vi "Estimate_State-Space_Model_from_FRFs_Parameter_Adjustment_v3.vi"() -> ()   [LabVIEW 2022 SP3]
doc: "This example demonstrates how to use frequency-domain data to estimate a state-space model. \n\n<B>Instructions:</B>\n1) Run this VI.\n2) Observe how the simulated frequency response matches the measured frequency response.\n3) Change the orders of the models, and observe how these changes affect the estimation error."
uses:
  WhiteNoise.ctl
  <vilib>/addons/System Identification/Model Typedefs.llb/SI Pole-Zero Plot.ctl
  <vilib>/addons/System Identification/Frequency Domain Estimation.llb/SI Estimate Discrete State-Space Model from FRF (SISO Arbitrary).vi
  <vilib>/addons/System Identification/Model Analysis.llb/SI Model Simulation (SISO Waveform).vi
  <vilib>/measure/maspectr.llb/FFT Spectrum (Mag-Phase) for 1 Chan.vi
  <vilib>/addons/System Identification/NI_SysID.lvlib
  <vilib>/addons/System Identification/Model Management Subs.llb/SI Get Order of SS Model (SISO).vi
  <vilib>/measure/NI_MABase.lvlib
  <vilib>/measure/NI_MAPro.lvlib
panel:
  out "Phase 2":cluster{"f0":dbl, "df":dbl, "phase":dbl[]}(graph)
  out "Mag 2":cluster{"f0":dbl, "df":dbl, "magnitude":dbl[]}(graph)
  out "Waveform Graph 2":waveform(dbl)(graph)
  out "Waveform Graph":waveform(dbl)(graph)
  in  "?":enum32{"White Noise", "Harmonic"}(tab)
  in  "Cluster":T2={"Seed"=0.0, "Standard Deviation"=0.2, "Reset"=FALSE, "Iterator"=1.0} {"Standard Deviation" format="%0.2p"}
  in  "Cluster 2":T3={"Iterator"=1.0, "Waveform Type"=0, "Frequency"=10.0, "Amplitude"=0.5} {"Frequency" format="%0.2p"; "Waveform Type" items=["Sine Wave", "Triangle Wave", "Square Wave", "Sawtooth Wave"]; "Amplitude" format="%0.2p"}
  out "sampling rate (Hz)":dbl
  out "model":picture
  out "number of states":i32
  out "Phase Error":cluster{dbl[], dbl[]}(graph)
  in  "confidence level (%)":dbl=99.0 format="%_2f"
  out "pole-zero plot":T4
  in  "name or relative path":path=path "C:/Users/LAV-UFSC/OneDrive - UFSC/Documents/LAV - TCC/Dados-Experimentos/25-04/frf_2.txt"
  in  "noise subspace (%)":dbl=78.0
  in  "FRF format":T5={"dB on? (F)"=FALSE, "unwrap phase? (F)"=FALSE, "convert to degree? (F)"=TRUE}
  out "Phase Response":cluster{"frequency":dbl[], "amplitude":dbl[]}[](graph)
  out "Magnitude Response":cluster{"frequency":dbl[], "amplitude":dbl[]}[](graph)
  in  "Order":i32=9
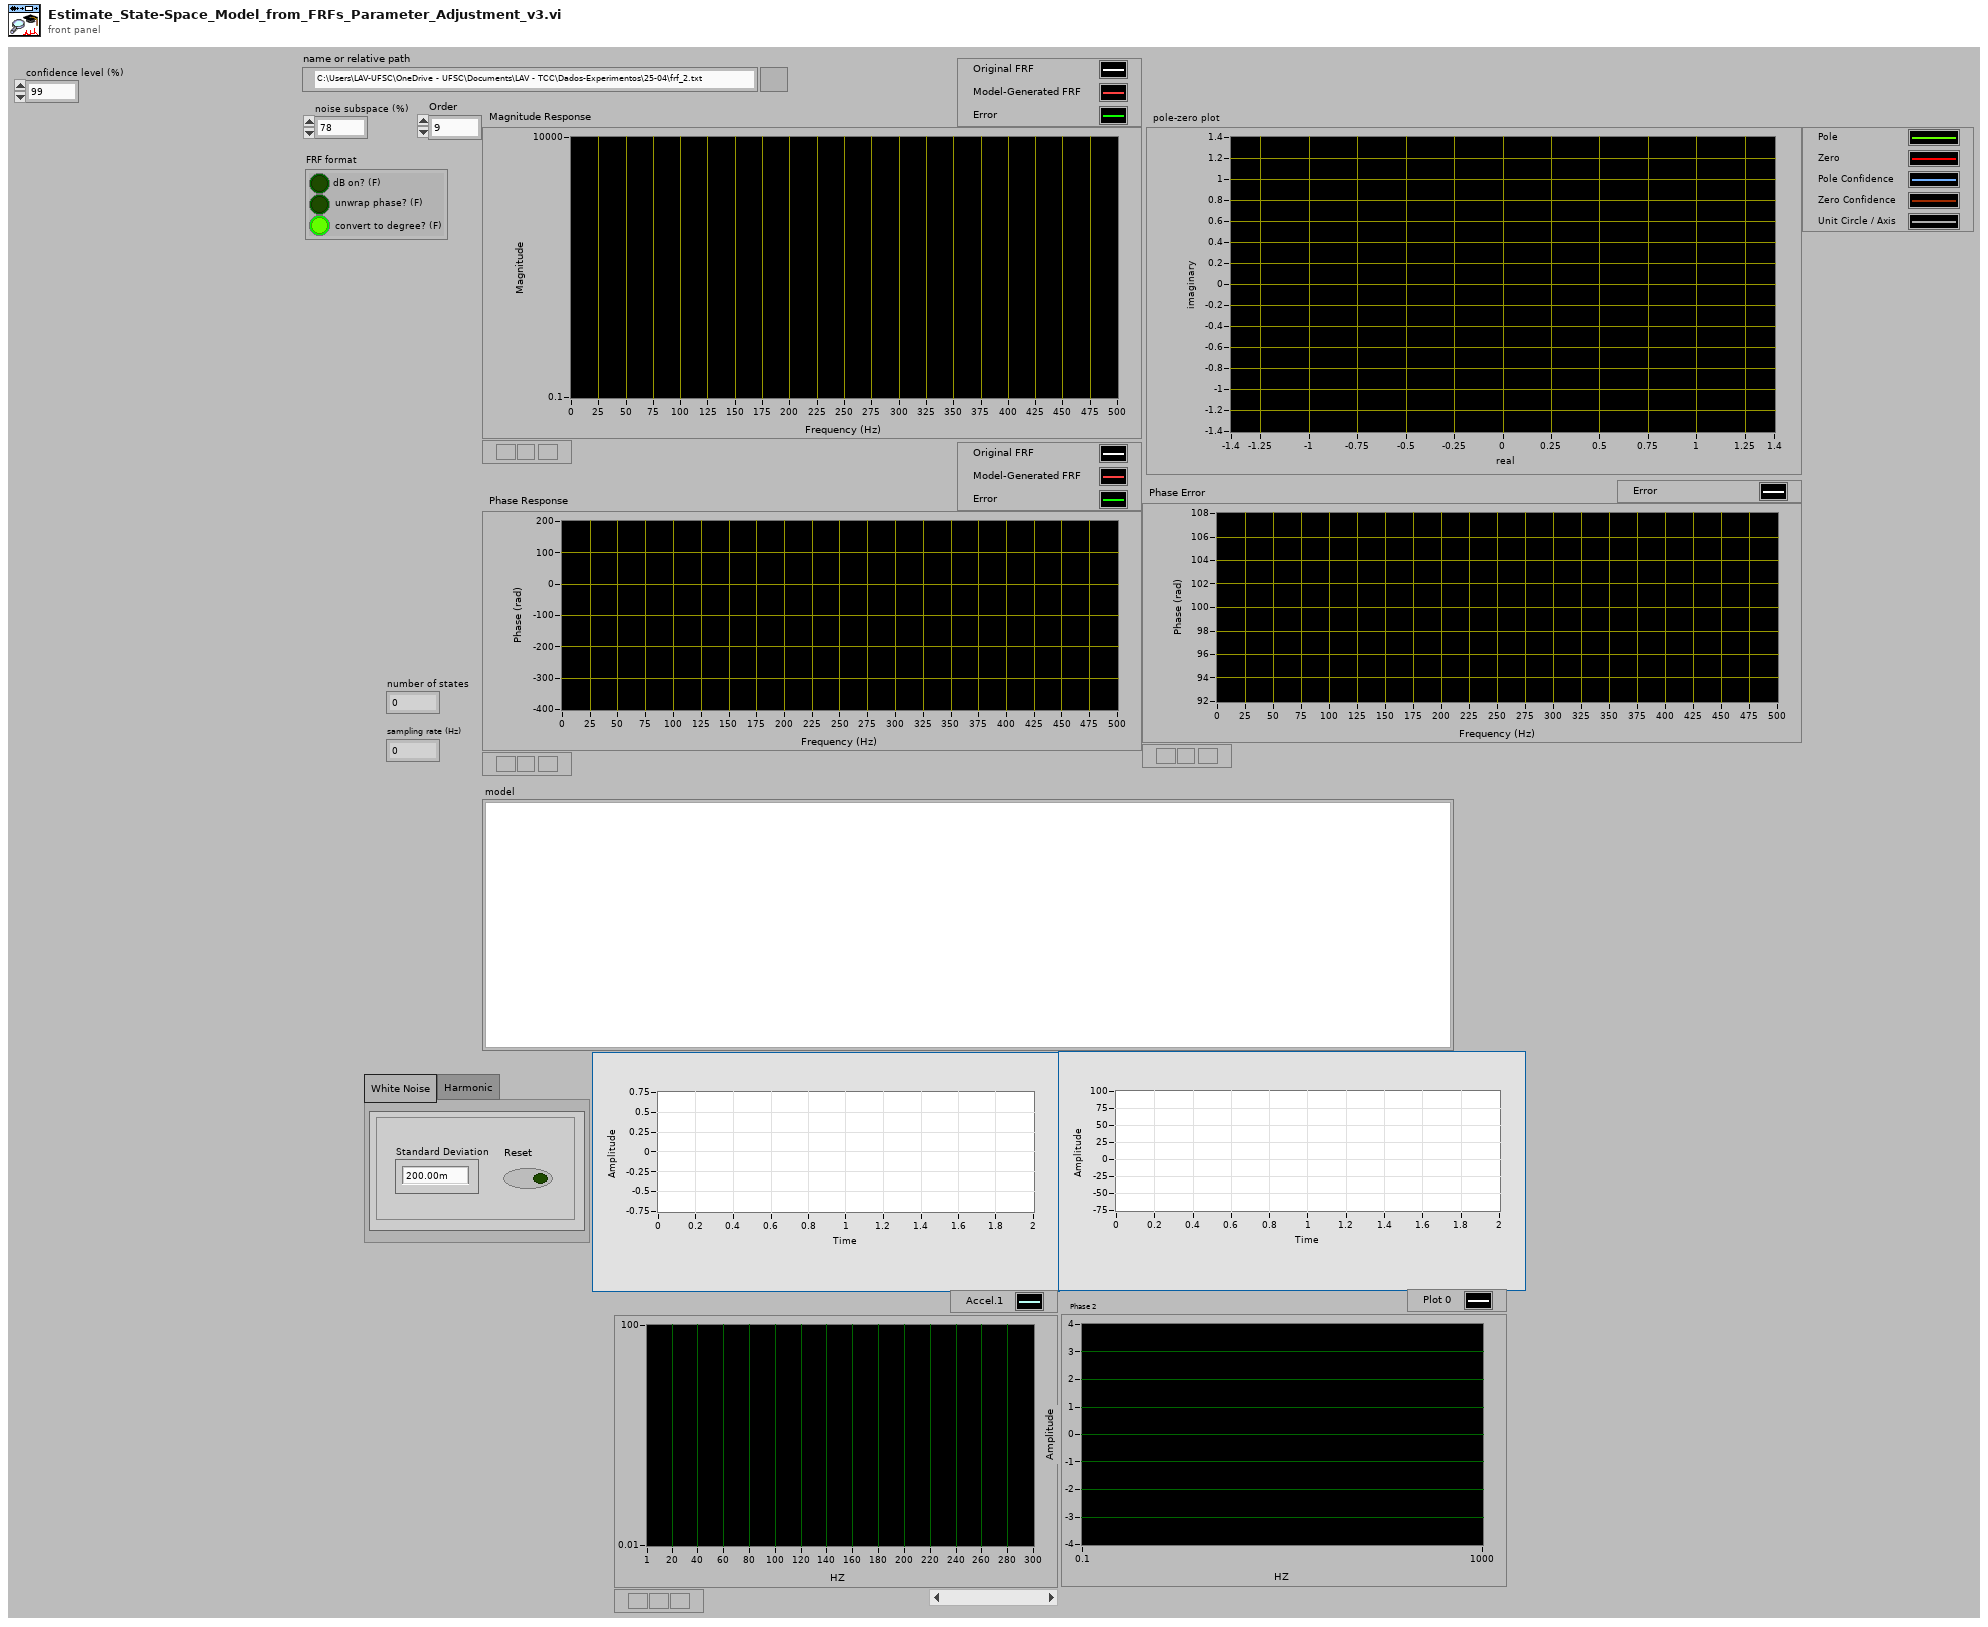
[diagram p1: front panel]
types:
  T1 = typedef "WhiteNoise.ctl" = dbl
  T2 = cluster{"Seed":T1, "Standard Deviation":dbl, "Reset":bool, "Iterator":dbl}
  T3 = cluster{"Iterator":dbl, "Waveform Type":u16, "Frequency":dbl, "Amplitude":dbl}
  T4 = typedef "NI_SysID.lvlib/SI Pole-Zero Plot.ctl" = cluster{"frequency":dbl[], "amplitude":dbl[]}[]
  T5 = cluster{"dB on? (F)":bool, "unwrap phase? (F)":bool, "convert to degree? (F)":bool}
  T6 = cluster{"start frequency":dbl, "end frequency":dbl, "num of freq bins":i32, "interval type":u16}
  T7 = typedef "NI_SysID.lvlib/si_generic model.ctl" = cluster{"attributes":cluster{"version":string, "model type":T8, "input names":string[], "output names":string[], "notes":string}, "coefficients":cluster{"A ":dbl[][][], "B":dbl[][][], "F":dbl[][][], "C":dbl[][][], "D":dbl[][][]}, "std deviations":cluster{"A ":dbl[][][], "B":dbl[][][], "F":dbl[][][], "C":dbl[][][], "D":dbl[][][]}, "coefficients covariance":dbl[][][], "noise variance":dbl[][], "fs":dbl, "system info":cluster{"number of inputs":i32, "number of outputs":i32, "A order":i32[][], "B order":i32[][], "F order":i32[][], "C order":i32[][], "D order":i32[][], "Delays":i32[][]}, "kalman gain":dbl[][], "initial state":dbl[], "trans func":cluster{"betas":dbl[], "alphas":dbl[]}[][], "zeros-poles":cluster{"zeros":cdb[], "poles":cdb[], "gain":dbl}[][], "std of trans func":cluster{"betas":dbl[], "alphas":dbl[]}[][], "std of zeros-poles":cluster{"zeros":cdb[], "poles":cdb[], "gain":dbl}[][], "trans func (noise)":cluster{"betas":dbl[], "alphas":dbl[]}[][], "std of trans func (noise)":cluster{"betas":dbl[], "alphas":dbl[]}[][], "zeros-poles (noise)":cluster{"zeros":cdb[], "poles":cdb[], "gain":dbl}[][], "std of zeros-poles (noise)":cluster{"zeros":cdb[], "poles":cdb[], "gain":dbl}[][], "Symbolic State Space Model":cluster{"Symbolic A":string[][], "Symbolic B":string[][], "Symbolic C":string[][], "Symbolic D":string[][], "Symbolic K":string[][], "Symbolic Initial State":string[]}, "delay":dbl[][], "variables":T9, "grey trans func spec":cluster{"orders of TF model":cluster{" num order":i32, "den order":i32}, "# of zeros/poles at origin":cluster{"zeros/poles":u16, "number ":i32}, "delay initial?":bool, "gain initial?":bool}}
  T8 = typedef "NI_SysID.lvlib/SI Model Type.ctl" = u16
  T9 = typedef "NI_SysID.lvlib/si_variables.ctl" = cluster{"name":string, "initial guess":dbl, "upper limit":dbl, "lower limit":dbl, "value":dbl}[]
  T10 = typedef "NI_SysID.lvlib/si_Bode Phase Plot.ctl" = cluster{"frequency":dbl[], "amplitude":dbl[]}[]
  T11 = typedef "NI_SysID.lvlib/si_Bode Magnitude Plot.ctl" = cluster{"frequency":dbl[], "amplitude":dbl[]}[]
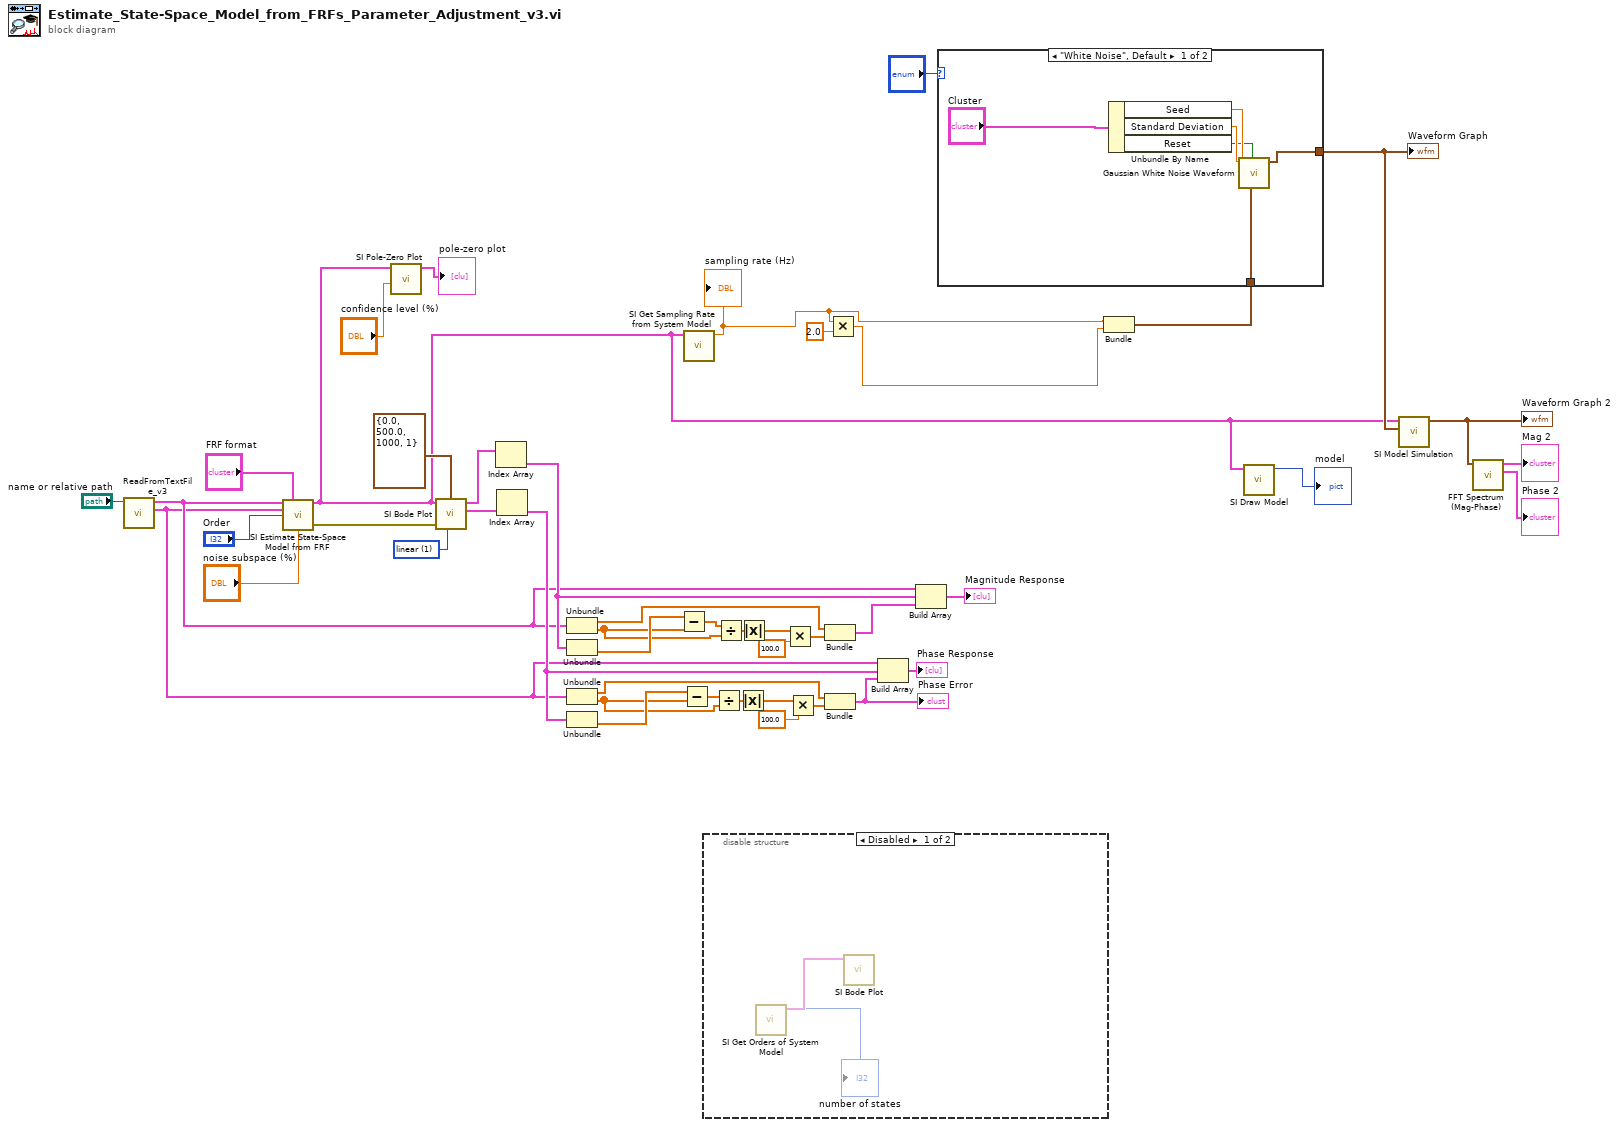
[diagram p0: block diagram]
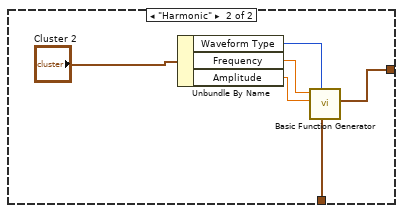
[diagram p2: hidden frame]
diagram:
  w38 = u16 1 items=["dB", "linear"] ("magnitude unit")
  n1 = call "ReadFromTextFile_v3.vi"("name or relative path"="name or relative path") -> ("Phase"=w20:cluster{dbl[], dbl[]}, "Magnitude"=w21:cluster{dbl[], dbl[]})  [unwired: 6 in, 2 out]
  n2 = call-poly <vilib>:"SI Estimate State-Space Model from FRF.vi"("FRF magnitude"=w21, "FRF format"="FRF format", "FRF phase"=w20, "number of states"="Order", "noise subspace (%)"="noise subspace (%)") -> ("system model out"=w4:T7, "error out"=w39:errorcluster)  [unwired: 3 in, 6 out]
  n3 = call <vilib>:"SI Pole-Zero Plot.vi"("confidence level (%)"="confidence level (%)", "system model"=w4) -> ("pole-zero plot"=→"pole-zero plot":T4)  [unwired: 8 in, 1 out]
  n4 = call <vilib>:"SI Bode Plot.vi"("magnitude unit"=w38, "freq info"=T6 {"start frequency"=0.0, "end frequency"=500.0, "num of freq bins"=1000, "interval type"=1}, "error in (no error)"=w39, "system model"=w4) -> ("Bode phase plot"=w34:T10, "Bode magnitude plot"=w35:T11)  [unwired: 3 in, 3 out]
  n5 = Index Array(array=w35) -> (element=w22:cluster{"frequency":dbl[], "amplitude":dbl[]})  [unwired: 1 in]
  n6 = Index Array(array=w34) -> (element=w33:cluster{"frequency":dbl[], "amplitude":dbl[]})  [unwired: 1 in]
  n7 = Unbundle(w21) -> (w30:dbl[], w31:dbl[])
  n8 = Unbundle(w22) -> ("amplitude"=w32:dbl[])  [unwired: 1 out]
  n9 = Unbundle(w20) -> (w12:dbl[], w23:dbl[])
  n10 = Unbundle(w33) -> ("amplitude"=w28:dbl[])  [unwired: 1 out]
  n11 = Subtract(x=w32, y=w31) -> (x-y=w26:dbl[])
  n12 = Subtract(x=w28, y=w23) -> (x-y=w24:dbl[])
  n13 = call <vilib>:"SI Get Sampling Rate from System Model.vi"("system model"=w4) -> ("sampling rate (Hz)"=w5:dbl)  [unwired: 9 in, 1 out]
  "sampling rate (Hz)" <- w5
  n14 = disable-structure shown="Disabled" {
    frame Disabled {
      n15 = call-poly <vilib>:"SI Get Orders of System Model.vi"() -> ("number of states"=→"number of states":i32, "system model"=w48:T7)  [unwired: 9 in, 1 out]
      n16 = call <vilib>:"SI Bode Plot.vi"("system model"=w48) -> ()  [unwired: 6 in, 5 out]
    }
    frame Enabled {
    }
  }
  n17 = Divide(x=w24, y=w23) -> (x/y=w25:dbl[])
  n18 = Divide(x=w26, y=w31) -> (x/y=w29:dbl[])
  n19 = Absolute Value(x=w25) -> (abs(x)=w13:dbl[])
  n20 = Absolute Value(x=w29) -> (abs(x)=w15:dbl[])
  n21 = Multiply(x=w15, y=100.0) -> (x*y=w18:dbl[])
  n22 = Multiply(x=w13, y=100.0) -> (x*y=w17:dbl[])
  n23 = Bundle(w30, w18) -> (w27:cluster{dbl[], dbl[]})  [unwired: 1 in]
  n24 = Bundle(w12, w17) -> (w19:cluster{dbl[], dbl[]})  [unwired: 1 in]
  "Phase Error" <- w19
  n25 = Multiply(x=w5, y=2.0) -> (x*y=w6:dbl)
  n26 = Build Array(w20, w33, w19) -> (→"Phase Response":cluster{"frequency":dbl[], "amplitude":dbl[]}[])
  n27 = Build Array(w21, w22, w27) -> (→"Magnitude Response":cluster{"frequency":dbl[], "amplitude":dbl[]}[])
  n28 = Bundle("sampling rate (Hz)"=w5, w6) -> (w9:cluster{"sampling rate (Hz)":dbl, dbl})  [unwired: 1 in]
  n29 = case shown="\"White Noise\", Default" "?" {
    tunnel: w9 -> [w53 w59]
    tunnel: [w49 w55] -> w8
    frame "White Noise", Default {
      n30 = Unbundle By Name("Cluster") -> ("Seed"=w52:T1, "Standard Deviation"=w51:dbl, "Reset"=w50:bool)
      n31 = call <vilib>:"Gaussian White Noise Waveform.vi"("sampling info"=w53, "reset signal"=w50, "seed"=w52, "standard deviation"=w51) -> ("signal out"=w49:waveform(dbl))  [unwired: 6 in, 1 out]
    }
    frame "Harmonic" {
      n32 = Unbundle By Name("Cluster 2") -> ("Waveform Type"=w58:u16, "Frequency"=w57:dbl, "Amplitude"=w56:dbl)
      n33 = call <vilib>:"Basic Function Generator.vi"("sampling info"=w59, "signal type"=w58, "amplitude"=w56, "frequency"=w57) -> ("signal out"=w55:waveform(dbl))  [unwired: 5 in, 2 out]
    }
  }
  "Waveform Graph" <- w8
  n34 = call <vilib>:"SI Draw Model.vi"("system model"=w4) -> ("model"=→"model":picture)  [unwired: 8 in, 2 out]
  n35 = call-poly <vilib>:"SI Model Simulation.vi"("stimulus signal"=w8, "system model"=w4) -> ("response"=w3:waveform(dbl))  [unwired: 7 in, 2 out]
  "Waveform Graph 2" <- w3
  n36 = call-poly <vilib>:"FFT Spectrum (Mag-Phase).vi"("time signal"=w3) -> ("phase"=→"Phase 2":cluster{"f0":dbl, "df":dbl, "phase":dbl[]}, "magnitude"=→"Mag 2":cluster{"f0":dbl, "df":dbl, "magnitude":dbl[]})  [unwired: 6 in, 3 out]
